vi "ABR-Read Average Waveforms.vi"(0 "Path":path, 11 "error in":errorcluster) -> (4 "Neural":dbl[][](array[numeric]), 6 "CM":dbl[][](array[numeric]), 10 "Metrics":dbl[][](array[numeric]), 15 "error out":errorcluster)   [LabVIEW 2020]
uses:
  epl-vi-lib/Utility VIs/Array Manipulation VIs/Array-Dimensions (2D).vi
  <vilib>/regexp/Match Regular Expression.xnode
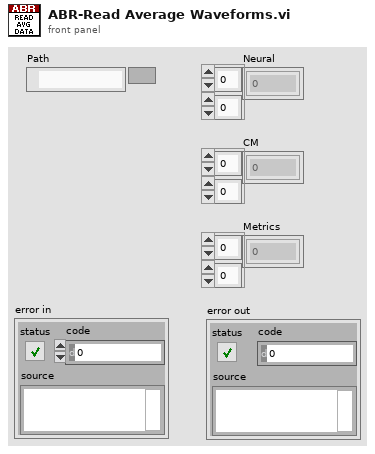
[diagram p1: front panel]
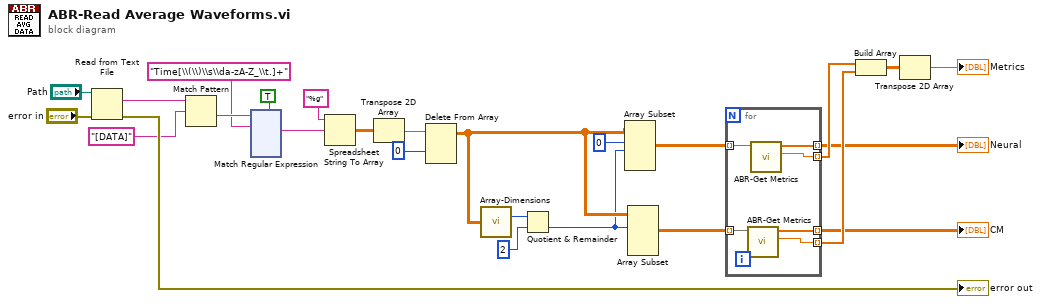
[diagram p0: block diagram]
diagram:
  n1 = Read from Text File(file (use dialog)="Path", error in="error in") -> (text=w2:string, error out=→"error out":errorcluster)  [unwired: 2 in, 2 out]
  n2 = Match Pattern(string=w2, regular expression="[DATA]" ("search string/char (-)")) -> (after substring=w25:string)  [unwired: 1 in, 3 out]
  n3 = xnode "Match Regular Expression"("input string"=w25, "regular expression"="Time[\\(\\)\\s\\da-zA-Z_\\t.]+", "multiline? (F)"=TRUE) -> ("after match"=w26:string)  [unwired: 3 in, 5 out]
  n4 = Spreadsheet String To Array(format string="%g" ("spreadsheet string"), spreadsheet string=w26) -> (array=w19:dbl[][])  [unwired: 2 in]
  n5 = Transpose 2D Array(2D array=w19) -> (transposed array=w20:dbl[][])
  n6 = Delete From Array(array=w20, index (row)=0 ("length")) -> (array with subset deleted=w22:dbl[][])  [unwired: 2 in, 1 out]
  n7 = call-poly "Array-Dimensions.vi"("2D Array"=w22) -> ("# rows"=w4:i32)  [unwired: 13 in, 1 out]
  n8 = Quotient & Remainder(x=w4, y=2) -> (floor(x/y)=w9:i32)  [unwired: 1 out]
  n9 = Array Subset(array=w22, index (row)=0 ("index"), length (row)=w9) -> (w7:dbl[][])  [unwired: 2 in]
  n10 = Array Subset(array=w22, index (row)=w9) -> (w8:dbl[][])  [unwired: 3 in]
  n11 = for {
    tunnel: w7 -> [w28] mode=indexing
    tunnel: w8 -> [w27] mode=indexing
    tunnel: [w32] -> w11 mode=indexing
    tunnel: [w31] -> w12 mode=indexing
    tunnel: [w30] -> w15 mode=indexing
    tunnel: [w29] -> w16 mode=indexing
    n12 = call "ABR-Get Metrics.vi"("Data in"=w27) -> ("spread value"=w29:dbl, "Data out"=w31:dbl[])  [unwired: 8 in, 1 out]
    n13 = call "ABR-Get Metrics.vi"("Data in"=w28) -> ("spread value"=w30:dbl, "Data out"=w32:dbl[])  [unwired: 8 in, 1 out]
  }
  "CM" <- w12
  "Neural" <- w11
  n14 = Build Array(w15, w16) -> (w13:dbl[][])
  n15 = Transpose 2D Array(2D array=w13) -> (transposed array=→"Metrics":dbl[][])
